vi "ErrorClusterEdit.vi"(10 "ErrorCode":i32, 11 "error in":errorcluster) -> (3 "error out":errorcluster)   [LabVIEW 2018]
panel:
  # "<機能>\nErrorクラスタのcodeとsourceを書き換える。"
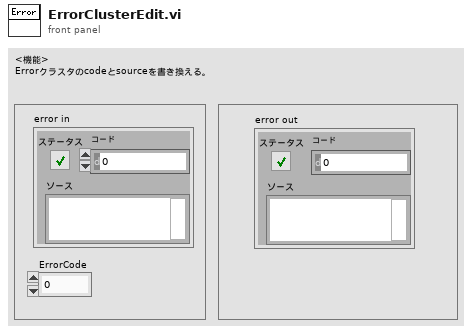
[diagram p1: front panel]
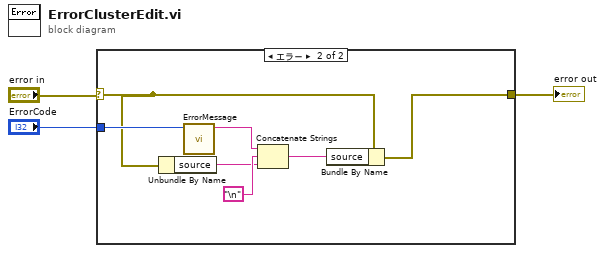
[diagram p0: block diagram]
diagram:
  n1 = case shown="エラー" "error in" {
    selector: "error in" -> [w4 w9]
    tunnel: [w4 w11] -> w2
    tunnel: "ErrorCode" -> [_ w10]
    frame No Error {
    }
    frame Error {
      n2 = Unbundle By Name(w9) -> ("source"=w6:string)
      n3 = call "ErrorMessage.vi"("ErrorCode"=w10) -> ("Message"=w8:string)  [unwired: 10 in]
      n4 = Concatenate Strings(w8, "\n", w6) -> (w5:string)
      n5 = Bundle By Name(cluster=w9, "source"=w5) -> (w11:errorcluster)
    }
  }
  "error out" <- w2
